vi "One Of.vi"(8 "error in (no error)":errorcluster, 11 "Mock in":refnum<class "Mock.lvclass">) -> (0 "error out":errorcluster, 3 "Mock out":refnum<class "Mock.lvclass">)   [LabVIEW 2020, in "One Of.lvclass"]
uses:
  One Of/One Of.lvclass
  Mock.lvclass
  C:/git/astemes-lmock/sandbox/Expectation/Expectation.lvclass
  One Of/One Of.lvclass/One Of.ctl
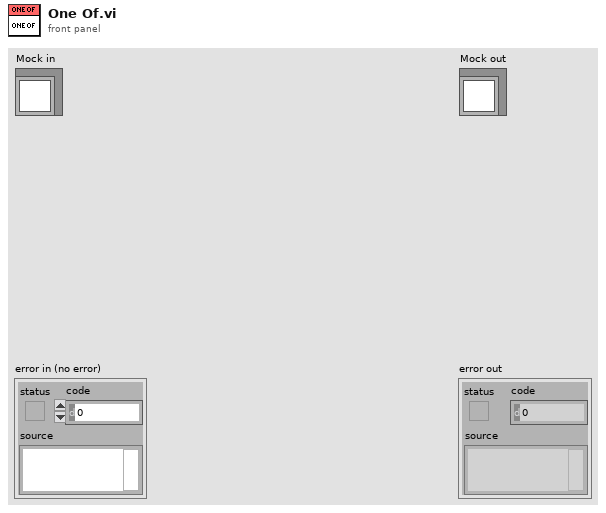
[diagram p1: front panel]
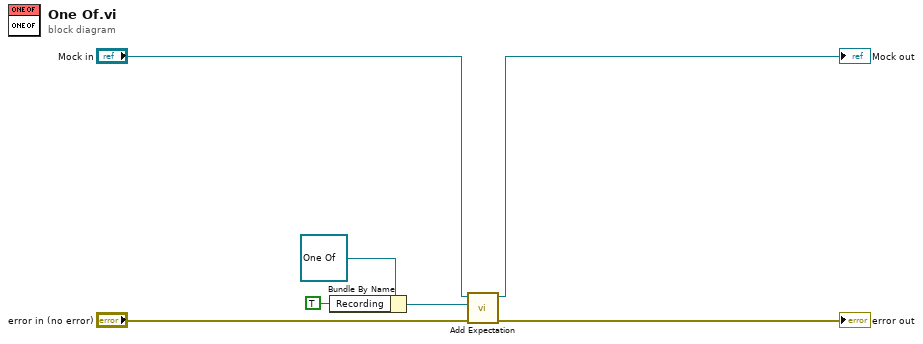
[diagram p0: block diagram]
diagram:
  n1 = Bundle By Name(cluster=refnum<class "One Of.lvclass"> refnum ("One Of.lvclass"), "Recording"=TRUE) -> (w2:refnum<class "One Of.lvclass">)
  n2 = call "Add Expectation.vi"("error in (no error)"="error in (no error)", "Expectations"=w2, "Mock in"="Mock in") -> ("error out"=→"error out":errorcluster, "Mock out"=→"Mock out":refnum<class "Mock.lvclass">)  [unwired: 7 in]
